vi "Initialize DAQ.vi"(8 "error in (no error)":errorcluster, 11 "Data in":T1) -> (0 "error out":errorcluster, 3 "Data out":T1)   [LabVIEW 2016, in "Acquisition.lvlib"]
uses:
  Acquisition.lvlib
  <vilib>/DAQmx/create/channels.llb/DAQmx Create Channel (AI-Voltage-Basic).vi
  <vilib>/DAQmx/create/channels.llb/DAQmx Create Channel (AO-Voltage-Basic).vi
  <vilib>/DAQmx/create/channels.llb/DAQmx Create Channel (CO-Pulse Generation-Time).vi
  <vilib>/DAQmx/configure/timing.llb/DAQmx Timing (Sample Clock).vi
  <vilib>/DAQmx/configure/timing.llb/DAQmx Timing (Implicit).vi
  <resource>/objmgr/daqmx.rc
  Data.ctl
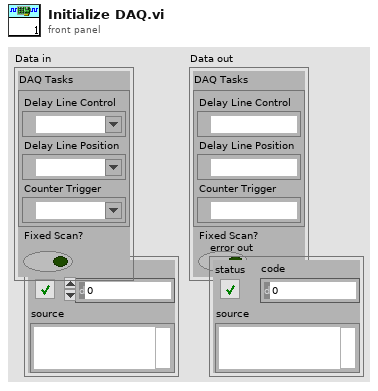
[diagram p1: front panel]
types:
  T1 = typedef "Data.ctl" = cluster{"DAQ Tasks":cluster{"Delay Line Control":refnum<k21>, "Delay Line Position":refnum<k21>, "Counter Trigger":refnum<k21>}, "Fixed Scan?":bool}
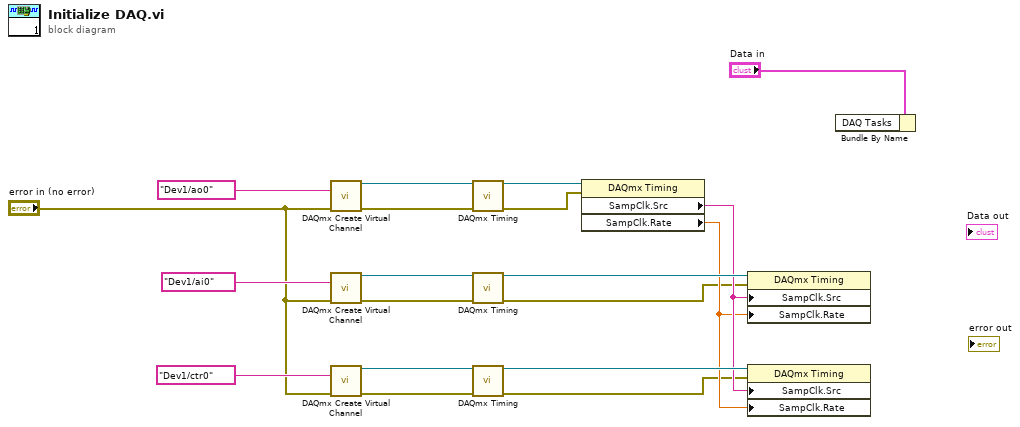
[diagram p0: block diagram]
diagram:
  n1 = call-poly <vilib>:"DAQmx Create Virtual Channel.vi"("physical channels"=tag "Dev1/ao0", "error in"="error in (no error)") -> ("task out"=w15:refnum<k21>, "error out"=w14:errorcluster)  [unwired: 12 in]
  n2 = call-poly <vilib>:"DAQmx Create Virtual Channel.vi"("physical channels"=tag "Dev1/ai0", "error in"="error in (no error)") -> ("task out"=w13:refnum<k21>, "error out"=w12:errorcluster)  [unwired: 12 in]
  n3 = call-poly <vilib>:"DAQmx Create Virtual Channel.vi"("counter"=tag "Dev1/ctr0", "error in"="error in (no error)") -> ("task out"=w10:refnum<k21>, "error out"=w11:errorcluster)  [unwired: 12 in]
  n4 = call-poly <vilib>:"DAQmx Timing.vi"("task/channels in"=w15, "error in"=w14) -> ("task out"=w9:refnum<k21>, "error out"=w2:errorcluster)  [unwired: 12 in]
  n5 = call-poly <vilib>:"DAQmx Timing.vi"("task/channels in"=w13, "error in"=w12) -> ("task out"=w8:refnum<k21>, "error out"=w4:errorcluster)  [unwired: 12 in]
  n6 = call-poly <vilib>:"DAQmx Timing.vi"("task/channels in"=w10, "error in"=w11) -> ("task out"=w7:refnum<k21>, "error out"=w3:errorcluster)  [unwired: 12 in]
  n7 = property class="DAQmx Timing"(reference=w9, error in=w2) -> ("SampClk.Src"=w6:tag, "SampClk.Rate"=w5:dbl)  [unwired: 2 out]
  n8 = property class="DAQmx Timing"(reference=w8, error in=w4, "SampClk.Src"=w6, "SampClk.Rate"=w5) -> ()  [unwired: 2 out]
  n9 = property class="DAQmx Timing"(reference=w7, error in=w3, "SampClk.Src"=w6, "SampClk.Rate"=w5) -> ()  [unwired: 2 out]
  n10 = Bundle By Name(cluster="Data in") -> ()  [unwired: 1 in, 1 out]
